vi "motorPos monitor.vi"() -> ()   [LabVIEW 2011]
uses:
  GUI_Template/GUI_master/tcp_new_data_event.ctl
  GUI_Template/GUI_master/tcp new data cluster.ctl
panel:
  out "Intensity Graph":dbl[][](graph)
  out "Numeric":i32
  in  "stop":bool
  out "Array":dbl[](array[numeric])
  in  "GUIdevice 99":string="PicoPad3"
  out "Waveform Graph":dbl[](graph)
  out "tcp data event":T1
  in  "Position.Axis 111::99":dbl=77.0 caption="Motor Axis 1" min=-20000.0 max=20000.0 format="%#_6f"
  in  "Position.Axis 112::99":dbl=77.0 caption="Motor Axis 1" min=-20000.0 max=20000.0 format="%#_6f"
  in  "Position.Axis 113::99":dbl=77.0 caption="Motor Axis 1" min=-20000.0 max=20000.0 format="%#_6f"
  in  "Position.Axis 121::99":dbl=77.0 caption="Motor Axis 1" min=-20000.0 max=20000.0 format="%#_6f"
  in  "Position.Axis 122::99":dbl=77.0 caption="Motor Axis 1" min=-20000.0 max=20000.0 format="%#_6f"
  in  "Position.Axis 123::99":dbl=77.0 caption="Motor Axis 1" min=-20000.0 max=20000.0 format="%#_6f"
  in  "Position.Axis 131::99":dbl=77.0 caption="Motor Axis 1" min=-20000.0 max=20000.0 format="%#_6f"
  in  "Position.Axis 132::99":dbl=77.0 caption="Motor Axis 1" min=-20000.0 max=20000.0 format="%#_6f"
  in  "Position.Axis 133::99":dbl=77.0 caption="Motor Axis 1" min=-20000.0 max=20000.0 format="%#_6f"
  in  "Position.Axis 141::99":dbl=77.0 caption="Motor Axis 1" min=-20000.0 max=20000.0 format="%#_6f"
  in  "Position.Axis 142::99":dbl=77.0 caption="Motor Axis 1" min=-20000.0 max=20000.0 format="%#_6f"
  in  "Position.Axis 143::99":dbl=77.0 caption="Motor Axis 1" min=-20000.0 max=20000.0 format="%#_6f"
  in  "Position.Axis 211::99":dbl=77.0 caption="Motor Axis 1" min=-20000.0 max=200000.0 format="%#_6f"
  in  "Position.Axis 212::99":dbl=77.0 caption="Motor Axis 1" min=-20000.0 max=20000.0 format="%#_6f"
  in  "Position.Axis 213::99":dbl=77.0 caption="Motor Axis 1" min=-20000.0 max=20000.0 format="%#_6f"
  in  "Position.Axis 221::99":dbl=77.0 caption="Motor Axis 1" min=-20000.0 max=20000.0 format="%#_6f"
  in  "Position.Axis 222::99":dbl=77.0 caption="Motor Axis 1" min=-20000.0 max=200000.0 format="%#_6f"
  in  "Position.Axis 223::99":dbl=77.0 caption="Motor Axis 1" min=-20000.0 max=20000.0 format="%#_6f"
  in  "Position.Axis 231::99":dbl=77.0 caption="Motor Axis 1" min=-20000.0 max=20000.0 format="%#_6f"
  in  "Position.Axis 232::99":dbl=77.0 caption="Motor Axis 1" min=-20000.0 max=20000.0 format="%#_6f"
  in  "Position.Axis 233::99":dbl=77.0 caption="Motor Axis 1" min=-20000.0 max=20000.0 format="%#_6f"
  in  "Position.Axis 241::99":dbl=77.0 caption="Motor Axis 1" min=-20000.0 max=20000.0 format="%#_6f"
  in  "Position.Axis 242::99":dbl=77.0 caption="Motor Axis 1" min=-20000.0 max=20000.0 format="%#_6f"
  in  "Position.Axis 243::99":dbl=77.0 caption="Motor Axis 1" min=-20000.0 max=20000.0 format="%#_6f"
  in  "Position.Axis 311::99":dbl=77.0 caption="Motor Axis 1" min=-20000.0 max=20000.0 format="%#_6f"
  in  "Position.Axis 312::99":dbl=77.0 caption="Motor Axis 1" min=-20000.0 max=20000.0 format="%#_6f"
  in  "Position.Axis 313::99":dbl=77.0 caption="Motor Axis 1" min=-999999.0 max=999999.0 format="%#_6f"
  in  "Position.Axis 321::99":dbl=77.0 caption="Motor Axis 1" min=-20000.0 max=20000.0 format="%#_6f"
  in  "Position.Axis 322::99":dbl=77.0 caption="Motor Axis 1" min=-20000.0 max=20000.0 format="%#_6f"
  in  "Position.Axis 323::99":dbl=77.0 caption="Motor Axis 1" min=-20000.0 max=20000.0 format="%#_6f"
  in  "Position.Axis 331::99":dbl=77.0 caption="Motor Axis 1" min=-20000.0 max=20000.0 format="%#_6f"
  in  "Position.Axis 332::99":dbl=77.0 caption="Motor Axis 1" min=-20000.0 max=20000.0 format="%#_6f"
  in  "Position.Axis 333::99":dbl=77.0 caption="Motor Axis 1" min=-20000.0 max=20000.0 format="%#_6f"
  in  "Position.Axis 341::99":dbl=77.0 caption="Motor Axis 1" min=-20000.0 max=20000.0 format="%#_6f"
  in  "Position.Axis 342::99":dbl=77.0 caption="Motor Axis 1" min=-20000.0 max=20000.0 format="%#_6f"
  in  "Position.Axis 343::99":dbl=77.0 caption="Motor Axis 1" min=-20000.0 max=20000.0 format="%#_6f"
  in  "Position.Axis 411::99":dbl=77.0 caption="Motor Axis 1" min=-20000.0 max=20000.0 format="%#_6f"
  in  "Position.Axis 412::99":dbl=77.0 caption="Motor Axis 1" min=-20000.0 max=20000.0 format="%#_6f"
  in  "Position.Axis 413::99":dbl=77.0 caption="Motor Axis 1" min=-20000.0 max=20000.0 format="%#_6f"
  in  "Position.Axis 421::99":dbl=77.0 caption="Motor Axis 1" min=-20000.0 max=20000.0 format="%#_6f"
  in  "Position.Axis 422::99":dbl=77.0 caption="Motor Axis 1" min=-20000.0 max=20000.0 format="%#_6f"
  in  "Position.Axis 423::99":dbl=77.0 caption="Motor Axis 1" min=-20000.0 max=20000.0 format="%#_6f"
  in  "Position.Axis 431::99":dbl=77.0 caption="Motor Axis 1" min=-20000.0 max=20000.0 format="%#_6f"
  in  "Position.Axis 432::99":dbl=77.0 caption="Motor Axis 1" min=-20000.0 max=20000.0 format="%#_6f"
  in  "Position.Axis 433::99":dbl=77.0 caption="Motor Axis 1" min=-20000.0 max=20000.0 format="%#_6f"
  in  "Position.Axis 441::99":dbl=77.0 caption="Motor Axis 1" min=-20000.0 max=20000.0 format="%#_6f"
  in  "Position.Axis 442::99":dbl=77.0 caption="Motor Axis 1" min=-20000.0 max=20000.0 format="%#_6f"
  in  "Position.Axis 443::99":dbl=77.0 caption="Motor Axis 1" min=-20000.0 max=20000.0 format="%#_6f"
  in  "Position.Axis 511::99":dbl=77.0 caption="Motor Axis 1" min=-20000.0 max=20000.0 format="%#_6f"
  in  "Position.Axis 512::99":dbl=77.0 caption="Motor Axis 1" min=-20000.0 max=20000.0 format="%#_6f"
  in  "Position.Axis 513::99":dbl=77.0 caption="Motor Axis 1" min=-20000.0 max=20000.0 format="%#_6f"
  in  "Position.Axis 521::99":dbl=77.0 caption="Motor Axis 1" min=-20000.0 max=20000.0 format="%#_6f"
  in  "Position.Axis 522::99":dbl=77.0 caption="Motor Axis 1" min=-20000.0 max=20000.0 format="%#_6f"
  in  "Position.Axis 523::99":dbl=77.0 caption="Motor Axis 1" min=-20000.0 max=20000.0 format="%#_6f"
  in  "Position.Axis 531::99":dbl=77.0 caption="Motor Axis 1" min=-20000.0 max=20000.0 format="%#_6f"
  in  "Position.Axis 532::99":dbl=77.0 caption="Motor Axis 1" min=-20000.0 max=20000.0 format="%#_6f"
  in  "Position.Axis 533::99":dbl=77.0 caption="Motor Axis 1" min=-20000.0 max=20000.0 format="%#_6f"
  in  "Position.Axis 541::99":dbl=77.0 caption="Motor Axis 1" min=-20000.0 max=20000.0 format="%#_6f"
  in  "Position.Axis 542::99":dbl=77.0 caption="Motor Axis 1" min=-20000.0 max=20000.0 format="%#_6f"
  in  "Position.Axis 543::99":dbl=77.0 caption="Motor Axis 1" min=-20000.0 max=20000.0 format="%#_6f"
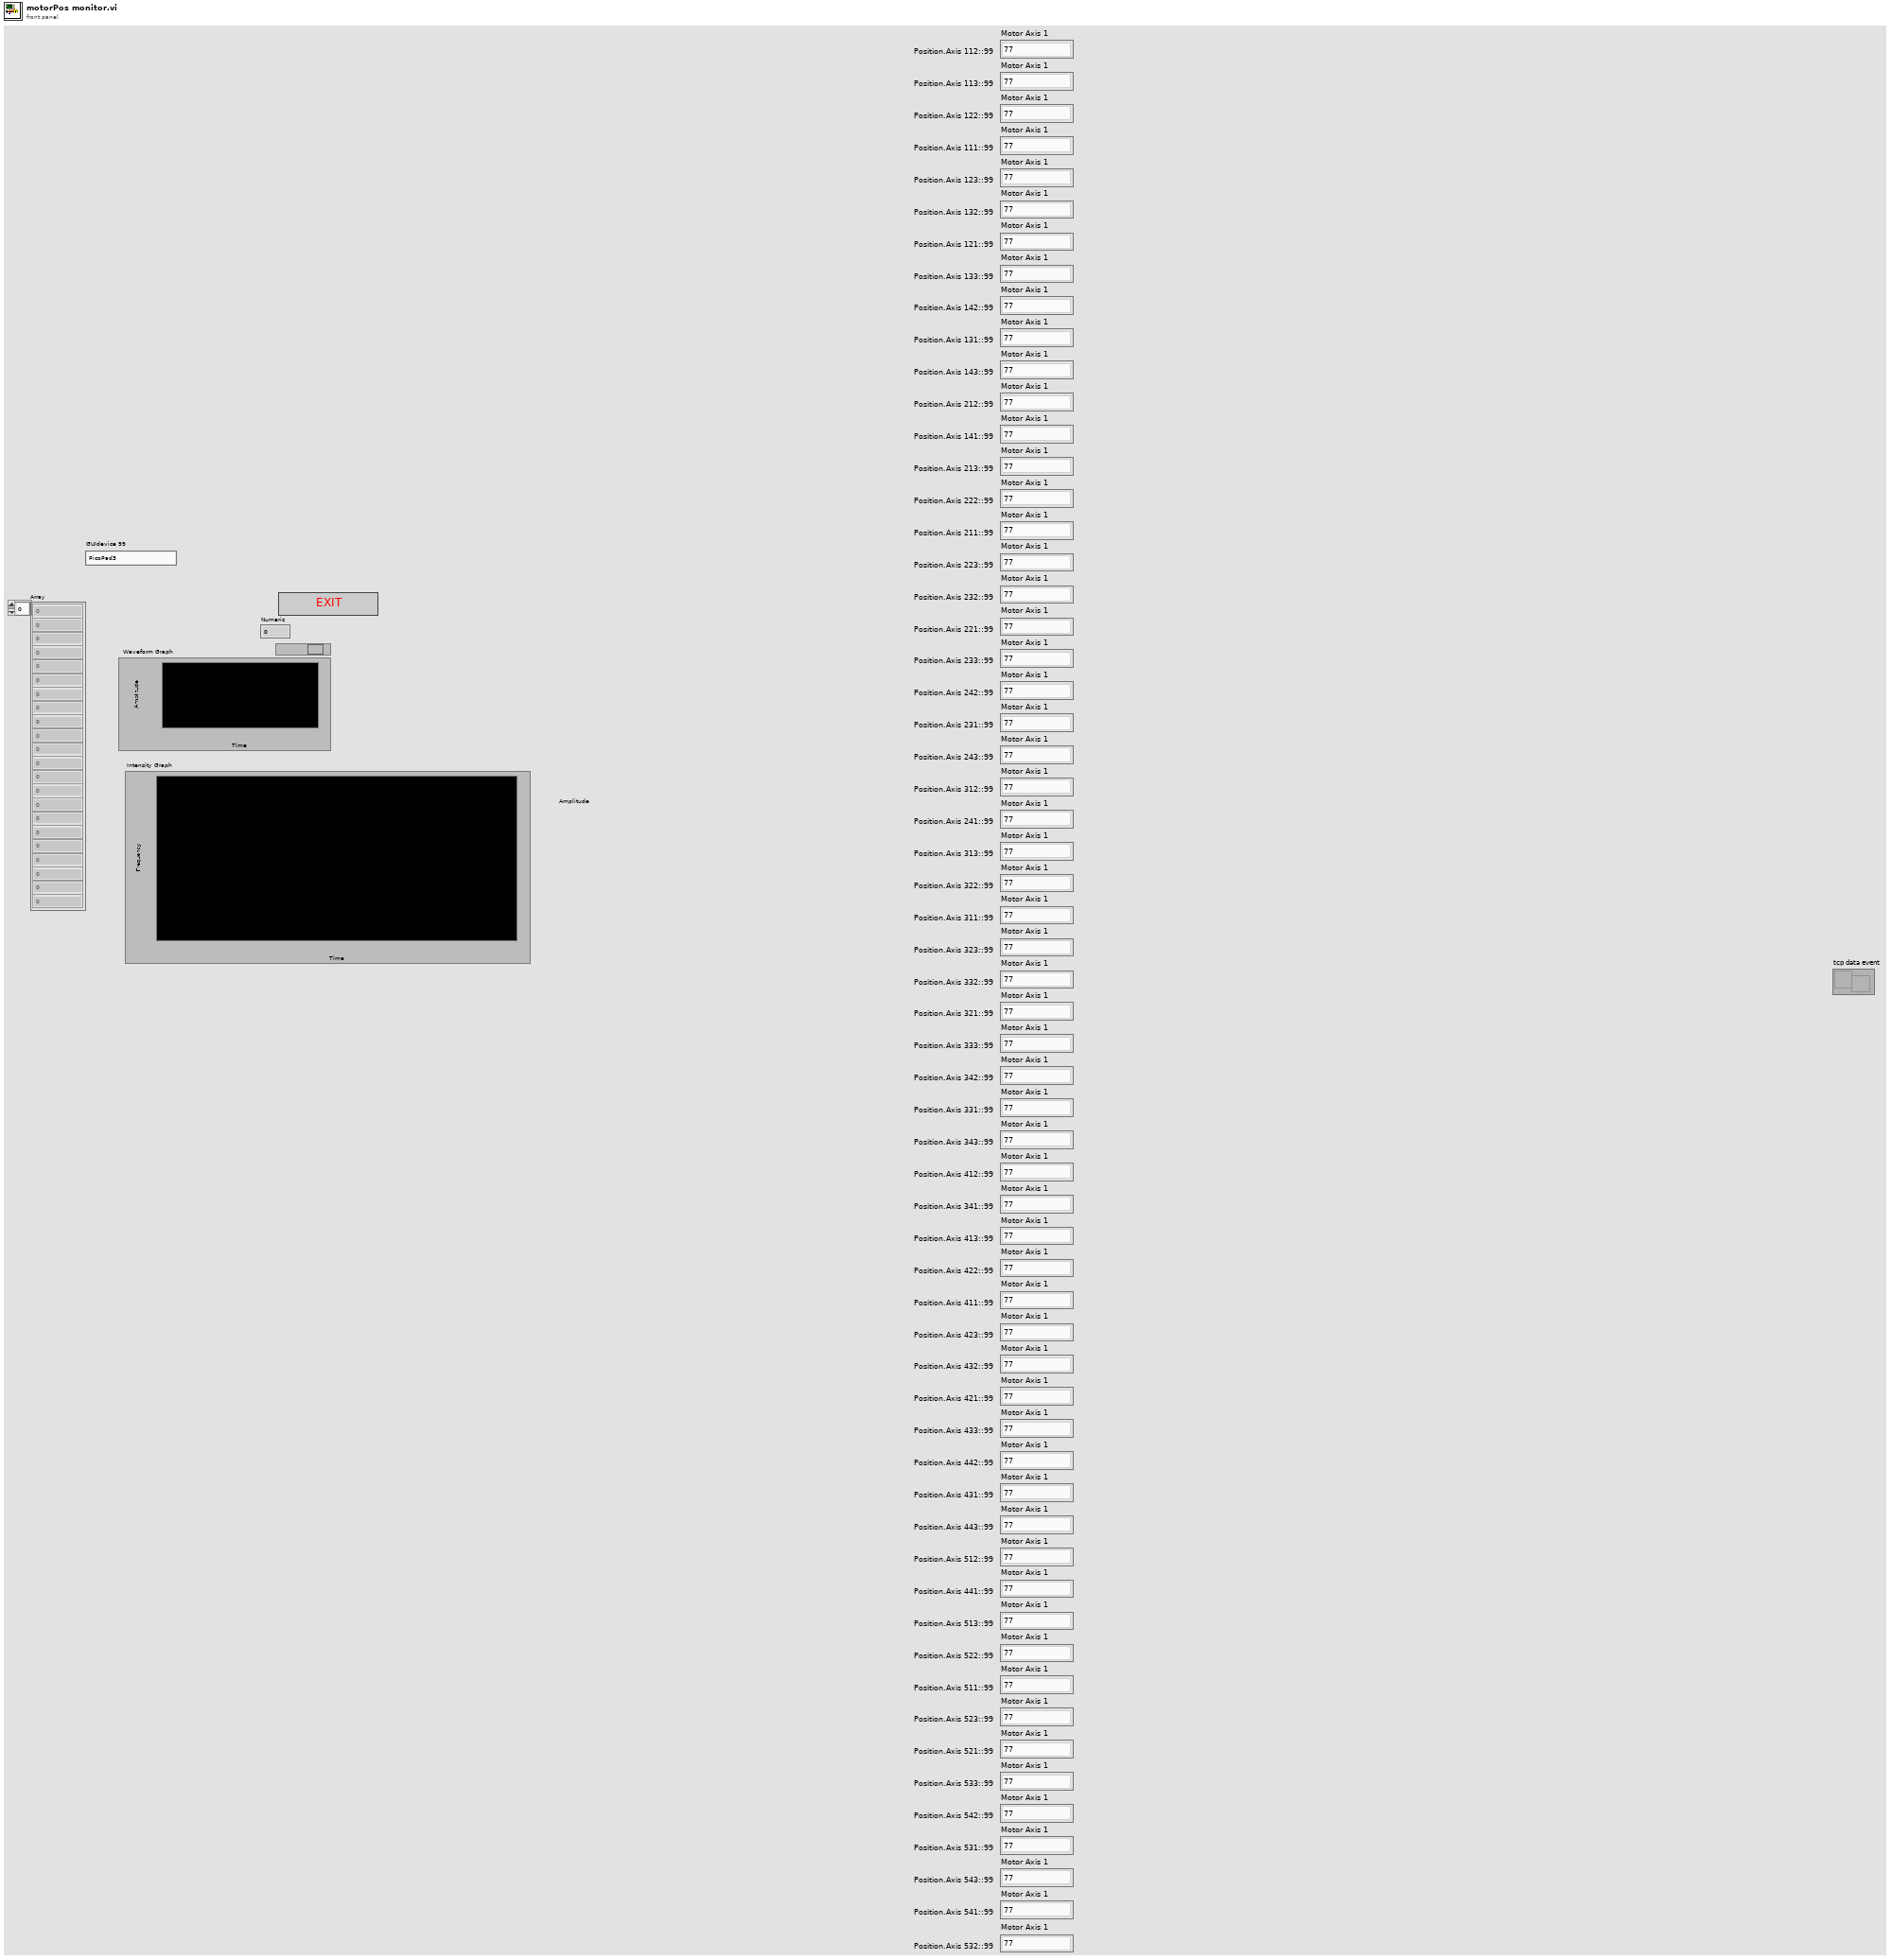
[diagram p1: front panel]
types:
  T1 = typedef "tcp_new_data_event.ctl" = refnum<user-event>
  T2 = typedef "tcp new data cluster.ctl" = cluster{"EventEnum":enum16{"new data", "connection status update"}, "Device name":string}
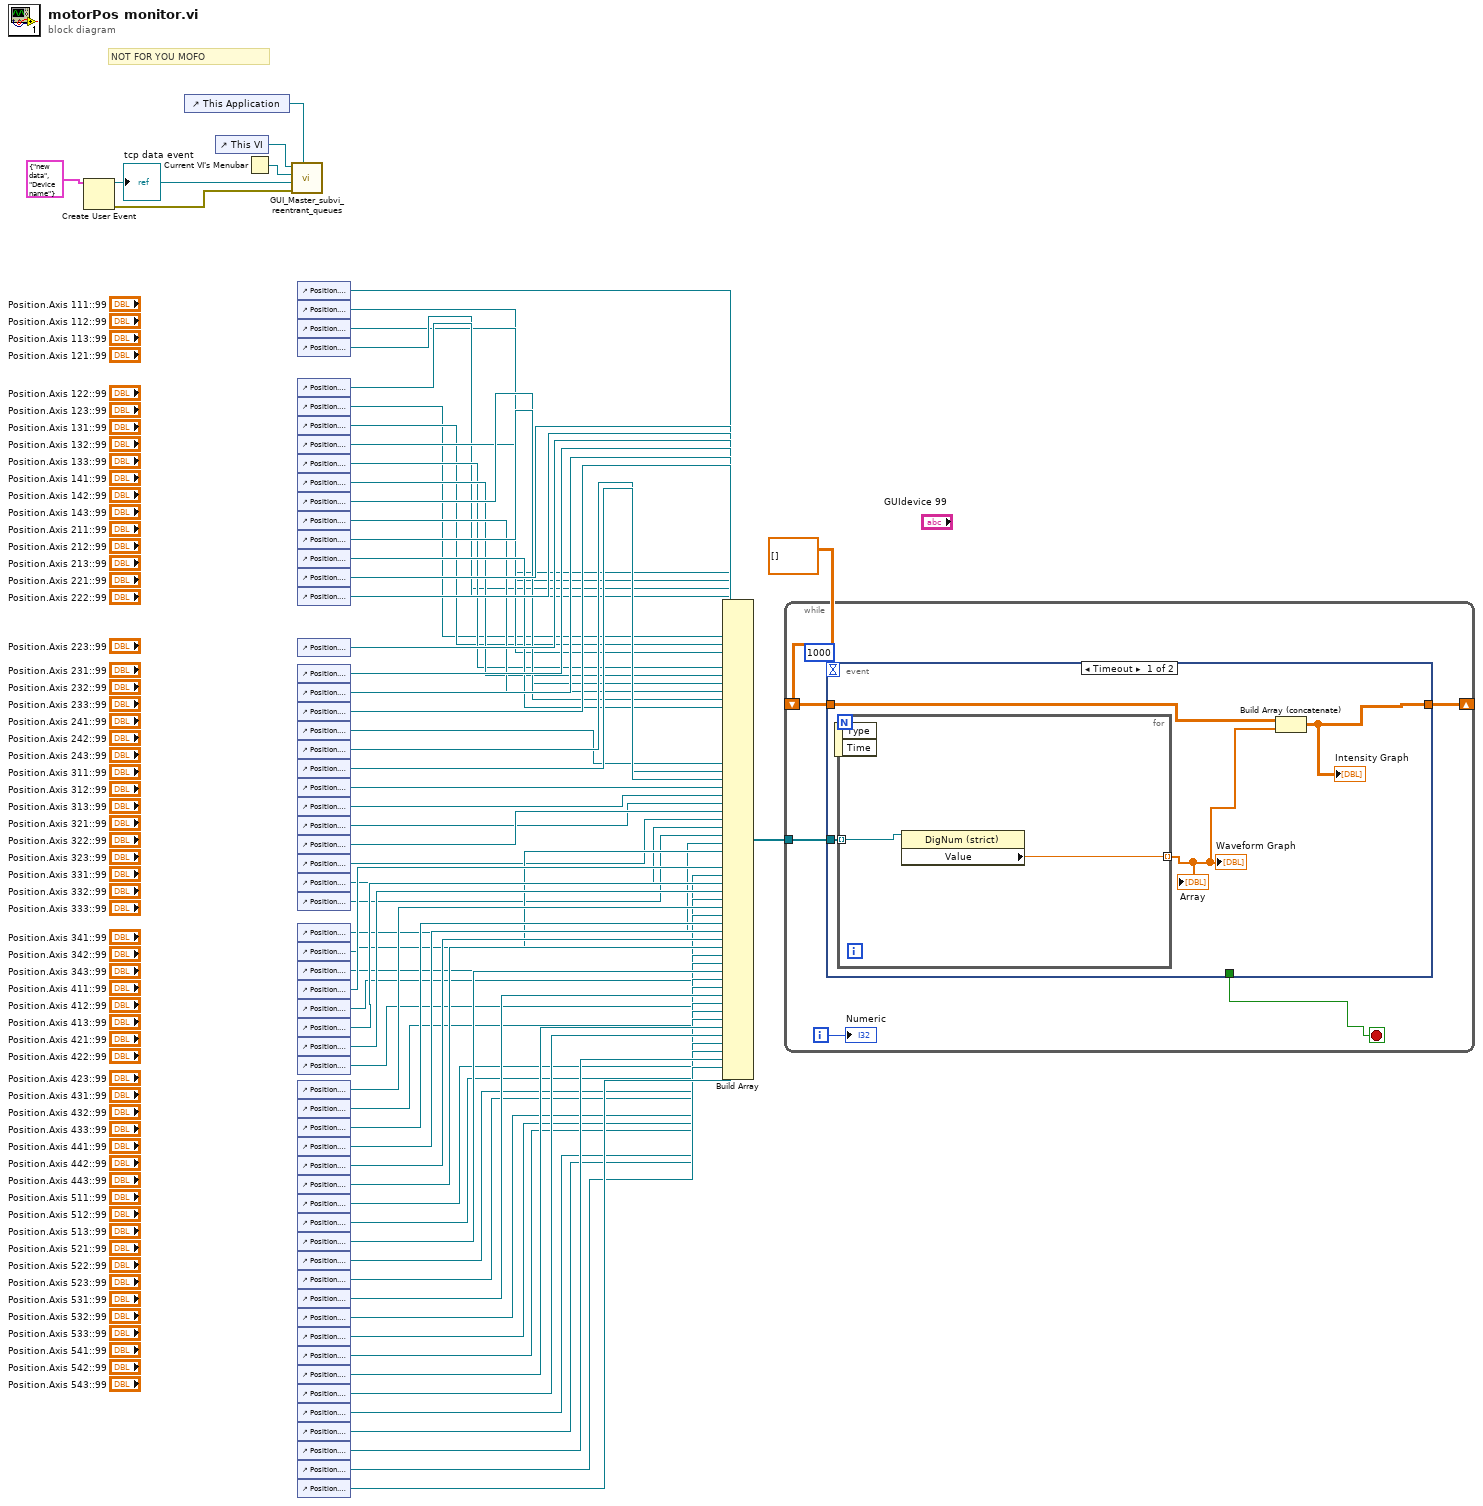
[diagram p0: block diagram]
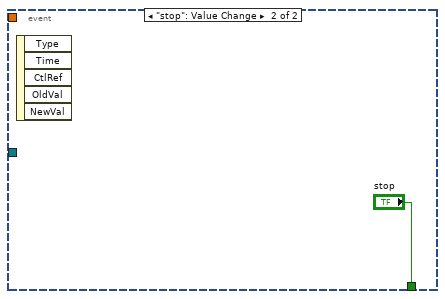
[diagram p2: hidden frame]
diagram:
  # "NOT FOR YOU MOFO"
  n1 = Create User Event(user event datatype=T2 {"EventEnum"=enum."new data", "Device name"="Device name"} ("New Event")) -> (user event=w8:refnum<user-event>, error out=w6:errorcluster)  [unwired: 1 in]
  "tcp data event" <- w8
  n2 = control-ref of="This Application"() -> (w7:refnum<vi>)
  n3 = control-ref of="This VI"() -> (w3:refnum<vi>)
  n4 = Current VI's Menubar() -> (w4:refnum<k9>)
  n5 = call "GUI_Master_subvi_reentrant_queues.vi"("This Application"=w7, "error in (no error)"=w6, "tcp data event"=w8, "Caller menu reference"=w4, "Caller VI ref"=w3) -> ()  [unwired: 6 in, 1 out]
  n6 = control-ref of="Position.Axis 111::99"() -> (w9:refnum<vi>)
  n7 = control-ref of="Position.Axis 112::99"() -> (w10:refnum<vi>)
  n8 = control-ref of="Position.Axis 113::99"() -> (w11:refnum<vi>)
  n9 = control-ref of="Position.Axis 121::99"() -> (w12:refnum<vi>)
  n10 = control-ref of="Position.Axis 122::99"() -> (w13:refnum<vi>)
  n11 = control-ref of="Position.Axis 123::99"() -> (w14:refnum<vi>)
  n12 = control-ref of="Position.Axis 131::99"() -> (w15:refnum<vi>)
  n13 = control-ref of="Position.Axis 132::99"() -> (w16:refnum<vi>)
  n14 = control-ref of="Position.Axis 133::99"() -> (w17:refnum<vi>)
  n15 = control-ref of="Position.Axis 141::99"() -> (w18:refnum<vi>)
  n16 = control-ref of="Position.Axis 142::99"() -> (w19:refnum<vi>)
  n17 = control-ref of="Position.Axis 143::99"() -> (w20:refnum<vi>)
  n18 = control-ref of="Position.Axis 211::99"() -> (w21:refnum<vi>)
  n19 = control-ref of="Position.Axis 212::99"() -> (w22:refnum<vi>)
  n20 = control-ref of="Position.Axis 213::99"() -> (w23:refnum<vi>)
  n21 = control-ref of="Position.Axis 221::99"() -> (w24:refnum<vi>)
  n22 = control-ref of="Position.Axis 222::99"() -> (w25:refnum<vi>)
  n23 = control-ref of="Position.Axis 223::99"() -> (w26:refnum<vi>)
  n24 = control-ref of="Position.Axis 231::99"() -> (w27:refnum<vi>)
  n25 = control-ref of="Position.Axis 232::99"() -> (w28:refnum<vi>)
  n26 = control-ref of="Position.Axis 233::99"() -> (w29:refnum<vi>)
  n27 = control-ref of="Position.Axis 241::99"() -> (w30:refnum<vi>)
  n28 = control-ref of="Position.Axis 242::99"() -> (w31:refnum<vi>)
  n29 = control-ref of="Position.Axis 243::99"() -> (w32:refnum<vi>)
  n30 = control-ref of="Position.Axis 311::99"() -> (w33:refnum<vi>)
  n31 = control-ref of="Position.Axis 312::99"() -> (w34:refnum<vi>)
  n32 = control-ref of="Position.Axis 313::99"() -> (w35:refnum<vi>)
  n33 = control-ref of="Position.Axis 321::99"() -> (w36:refnum<vi>)
  n34 = control-ref of="Position.Axis 322::99"() -> (w37:refnum<vi>)
  n35 = control-ref of="Position.Axis 323::99"() -> (w38:refnum<vi>)
  n36 = control-ref of="Position.Axis 331::99"() -> (w39:refnum<vi>)
  n37 = control-ref of="Position.Axis 332::99"() -> (w40:refnum<vi>)
  n38 = control-ref of="Position.Axis 333::99"() -> (w41:refnum<vi>)
  n39 = control-ref of="Position.Axis 341::99"() -> (w42:refnum<vi>)
  n40 = control-ref of="Position.Axis 342::99"() -> (w43:refnum<vi>)
  n41 = control-ref of="Position.Axis 343::99"() -> (w44:refnum<vi>)
  n42 = control-ref of="Position.Axis 411::99"() -> (w45:refnum<vi>)
  n43 = control-ref of="Position.Axis 412::99"() -> (w46:refnum<vi>)
  n44 = control-ref of="Position.Axis 413::99"() -> (w47:refnum<vi>)
  n45 = control-ref of="Position.Axis 421::99"() -> (w48:refnum<vi>)
  n46 = control-ref of="Position.Axis 422::99"() -> (w49:refnum<vi>)
  n47 = control-ref of="Position.Axis 423::99"() -> (w50:refnum<vi>)
  n48 = control-ref of="Position.Axis 431::99"() -> (w51:refnum<vi>)
  n49 = control-ref of="Position.Axis 432::99"() -> (w52:refnum<vi>)
  n50 = control-ref of="Position.Axis 433::99"() -> (w53:refnum<vi>)
  n51 = control-ref of="Position.Axis 441::99"() -> (w54:refnum<vi>)
  n52 = control-ref of="Position.Axis 442::99"() -> (w55:refnum<vi>)
  n53 = control-ref of="Position.Axis 443::99"() -> (w56:refnum<vi>)
  n54 = control-ref of="Position.Axis 511::99"() -> (w57:refnum<vi>)
  n55 = control-ref of="Position.Axis 512::99"() -> (w58:refnum<vi>)
  n56 = control-ref of="Position.Axis 513::99"() -> (w59:refnum<vi>)
  n57 = control-ref of="Position.Axis 521::99"() -> (w60:refnum<vi>)
  n58 = control-ref of="Position.Axis 522::99"() -> (w61:refnum<vi>)
  n59 = control-ref of="Position.Axis 523::99"() -> (w62:refnum<vi>)
  n60 = control-ref of="Position.Axis 531::99"() -> (w63:refnum<vi>)
  n61 = control-ref of="Position.Axis 532::99"() -> (w64:refnum<vi>)
  n62 = control-ref of="Position.Axis 533::99"() -> (w65:refnum<vi>)
  n63 = control-ref of="Position.Axis 541::99"() -> (w66:refnum<vi>)
  n64 = control-ref of="Position.Axis 542::99"() -> (w67:refnum<vi>)
  n65 = control-ref of="Position.Axis 543::99"() -> (w68:refnum<vi>)
  n66 = Build Array(w9, w10, w11, w12, w13, w14, w15, w16, w17, w18, w19, w20, w21, w22, w23, w24, w25, w26, w27, w28, w29, w30, w31, w32, w33, w34, w35, w36, w37, w38, w39, w40, w41, w42, w43, w44, w45, w46, w47, w48, w49, w50, w51, w52, w53, w54, w55, w56, w57, w58, w59, w60, w61, w62, w63, w64, w65, w66, w67, w68) -> (w2:refnum<vi>[])
  n67 = while {
    tunnel: w2 -> [w74]
    shift-right: [w71] -> _
    shift-left: dbl[][] [] -> [w72]
    i -> [w73]
    stop <- w69 stop-if-true
    n68 = event shown="[0] Timeout" {
      selector: _ -> [_ _]
      dyn-events: _ -> [_ _]
      timeout: 1000 -> [_ _]
      tunnel: w74 -> [w78 _]
      tunnel: w72 -> [w77 _]
      tunnel: [w75 _] -> w71
      tunnel: [_ "stop"] -> w69
      event Timeout {
        n69 = event-data() -> ()  [unwired: 1 in, 2 out]
        n70 = for {
          tunnel: w78 -> [w80] mode=indexing
          tunnel: [w79] -> w76 mode=indexing
          n71 = property class="DigNum (strict)"(reference=w80) -> ("Value"=w79:dbl)  [unwired: 1 in, 2 out]
        }
        "Waveform Graph" <- w76
        "Array" <- w76
        n72 = Build Array (concatenate)(w77, w76) -> (w75:dbl[][])
        "Intensity Graph" <- w75
      }
      event "stop": Value Change {
        n73 = event-data() -> ()  [unwired: 1 in, 5 out]
      }
    }
    "Numeric" <- w73
  }
